vi "Init tree for error log.vi"(8 "error in (no error)":errorcluster, 9 "Test Log(Schema)":string=" edcu_48v_thermal_endurance_test_dv_28_10_2024_19_48_44.error_log" caption="Test Log", 11 "TreeControl in":refnum<vi>) -> (0 "error out":errorcluster)   [LabVIEW 2023, in "Data Analysis.lvlib"]
uses:
  Data Analysis.lvlib
  HardwareAbstractionLayer_LVOOP/Database/Database.lvclass
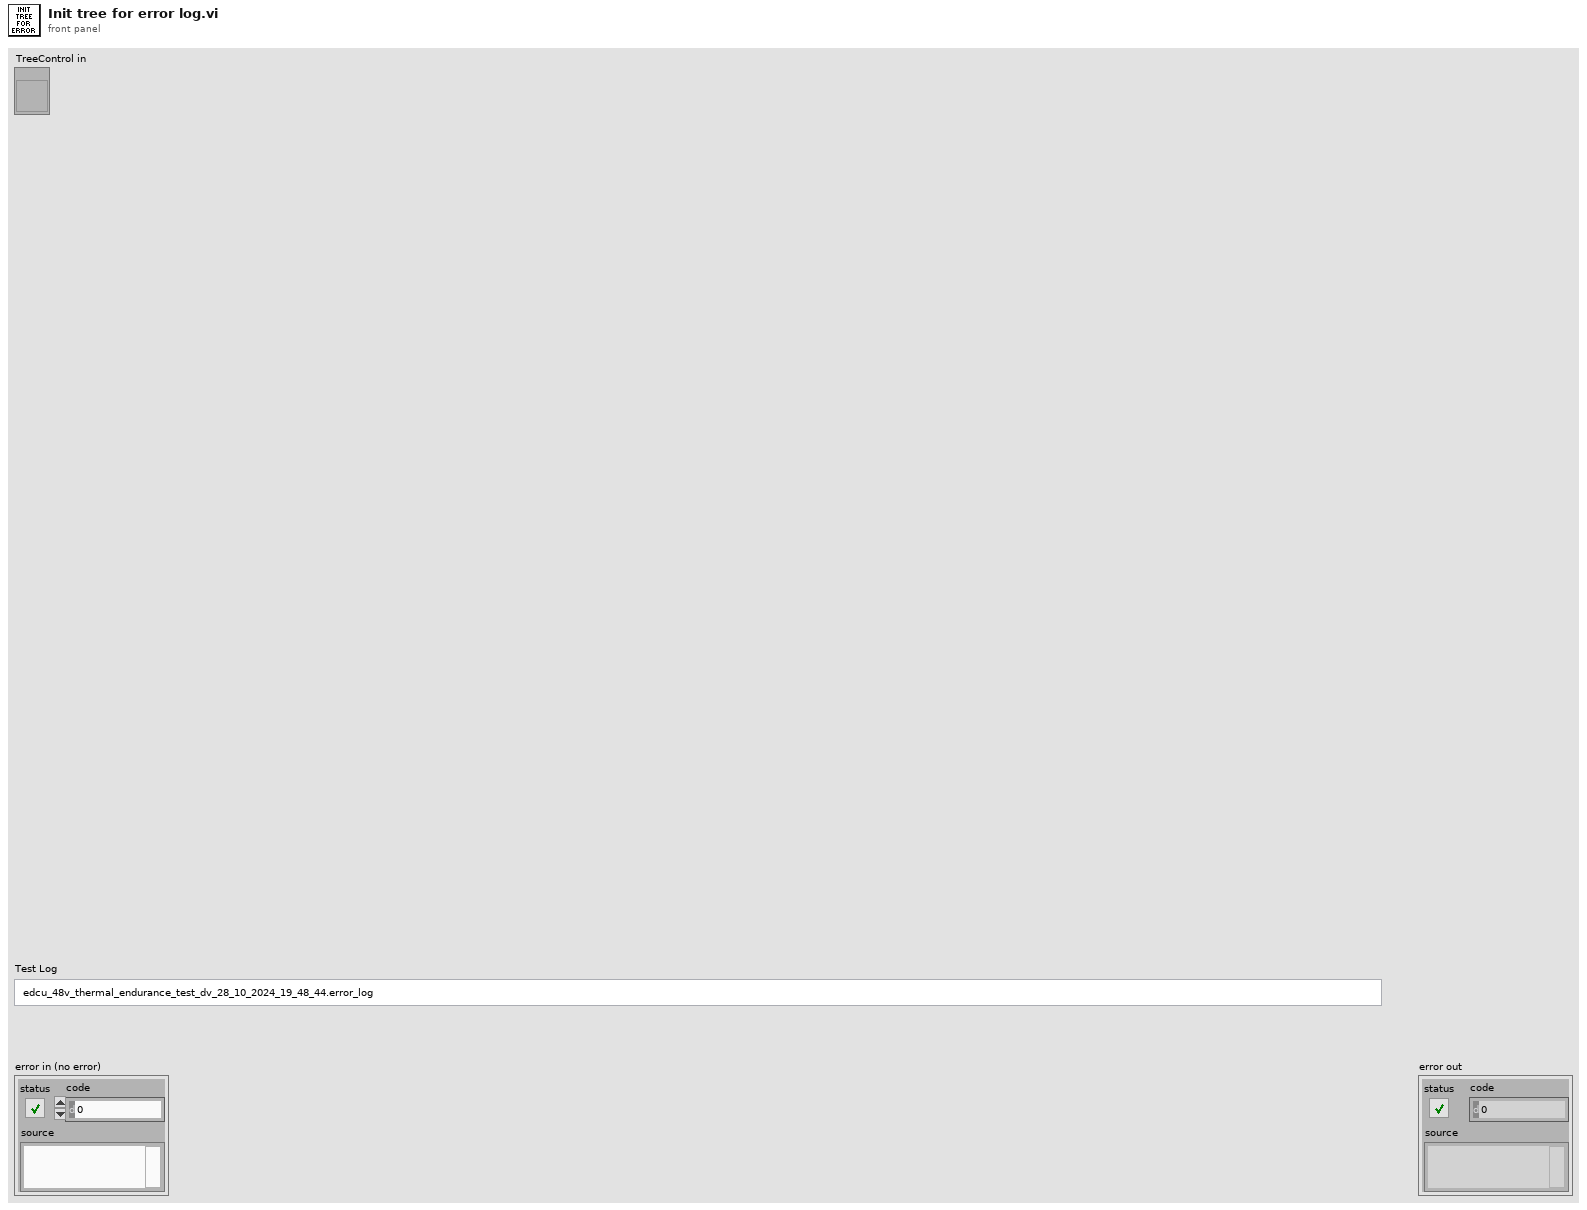
[diagram p1: front panel]
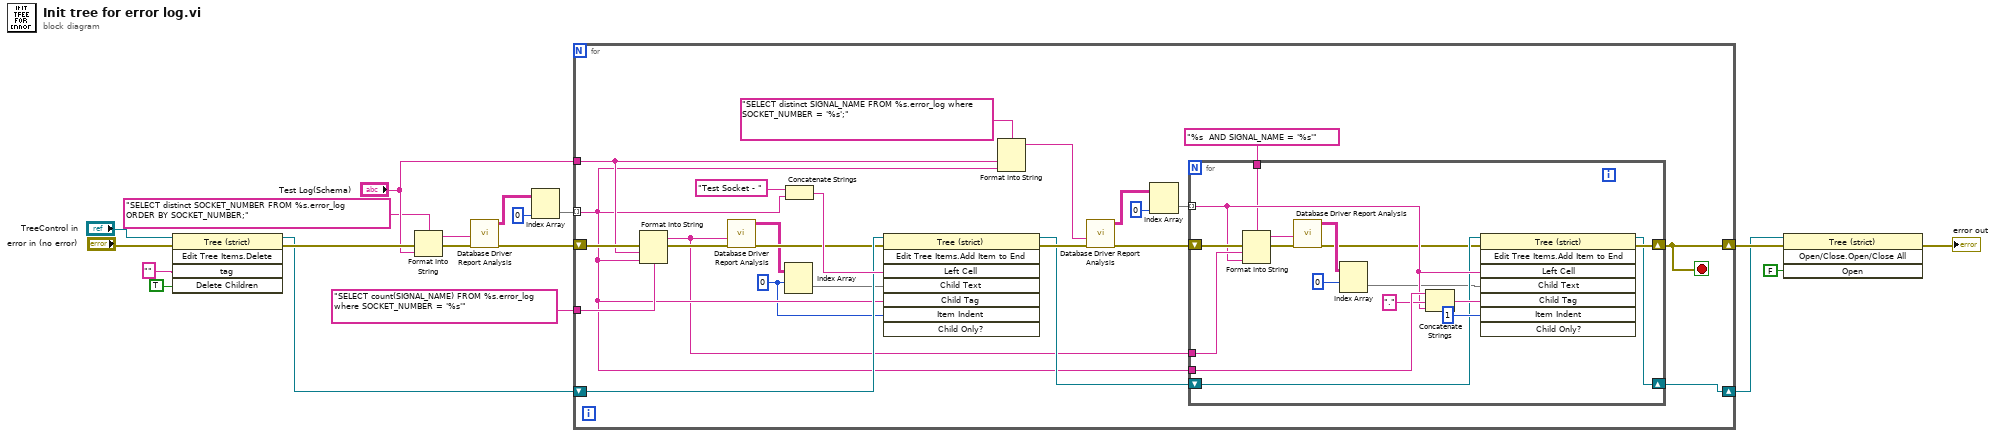
[diagram p0: block diagram]
diagram:
  n1 = invoke on="Invoke Node" class="Tree (strict)" method="Edit Tree Items.Delete"(reference="TreeControl in", error in="error in (no error)", "tag"="" ("Tag"), "Delete Children"=TRUE ("Delete Children?")) -> (reference out=w1:refnum<vi>, error out=w16:errorcluster)  [unwired: 1 in, 3 out]
  n2 = Format Into String(format string="SELECT distinct SOCKET_NUMBER FROM %s.error_log ORDER BY SOCKET_NUMBER;" ("SQL query"), error in=w16, "Test Log(Schema)") -> (resulting string=w12:string, error out=w17:errorcluster)  [unwired: 1 in]
  n3 = call "Database Driver Report Analysis.vi"("error in"=w17, "SQL query"=w12) -> ("error out"=w8:errorcluster, "data"=w9:string[][])  [unwired: 6 in, 2 out]
  n4 = Index Array(array=w9, index (col)=0 ("disabled index (col)")) -> (element=w10:string[])  [unwired: 1 in]
  n5 = for {
    tunnel: w10 -> [w25] mode=indexing
    shift-right: [w41] -> w18
    shift-left: w8 -> [w29]
    tunnel: "Test Log(Schema)" -> [w26]
    shift-right: [w31] -> w3
    shift-left: w1 -> [w33]
    tunnel: "SELECT count(SIGNAL_NAME) FROM %s.error_log where SOCKET_NUMBER = '%s'" ("SQL query") -> [w27]
    stop <- w41 stop-if-true
    w22 = 0 ("index (row)")
    n6 = Format Into String(format string=w27, error in=w29, w26, w25) -> (resulting string=w21:string, error out=w28:errorcluster)  [unwired: 1 in]
    n7 = call "Database Driver Report Analysis.vi"("error in"=w28, "SQL query"=w21) -> ("error out"=w30:errorcluster, "data"=w24:string[][])  [unwired: 6 in, 2 out]
    n8 = Index Array(array=w24, index (row)=w22) -> (element=w23:string[])  [unwired: 1 in]
    n9 = Concatenate Strings("Test Socket - " ("element"), w25) -> (w42:string)
    n10 = invoke on="Invoke Node" class="Tree (strict)" method="Edit Tree Items.Add Item to End"(reference=w33, error in=w30, "Left Cell"=w42, "Child Text"=w23, "Child Tag"=w25, "Item Indent"=w22) -> (reference out=w32:refnum<vi>, error out=w40:errorcluster)  [unwired: 2 in, 6 out]
    n11 = Format Into String(format string="SELECT distinct SIGNAL_NAME FROM %s.error_log where SOCKET_NUMBER = '%s';" ("SQL query"), w26, w25) -> (resulting string=w37:string)  [unwired: 2 in, 1 out]
    n12 = call "Database Driver Report Analysis.vi"("error in"=w40, "SQL query"=w37) -> ("error out"=w39:errorcluster, "data"=w35:string[][])  [unwired: 6 in, 2 out]
    n13 = Index Array(array=w35, index (col)=0 ("disabled index (col)")) -> (element=w34:string[])  [unwired: 1 in]
    n14 = for {
      shift-right: [w60] -> w41
      shift-left: w39 -> [w54]
      tunnel: w34 -> [w52] mode=indexing
      tunnel: w25 -> [w58]
      shift-right: [w55] -> w31
      shift-left: w32 -> [w50]
      tunnel: w21 -> [w53]
      tunnel: "%s  AND SIGNAL_NAME = '%s'" ("format string") -> [w51]
      n15 = Format Into String(format string=w51, error in=w54, w53, w52) -> (resulting string=w44:string, error out=w47:errorcluster)  [unwired: 1 in]
      n16 = call "Database Driver Report Analysis.vi"("error in"=w47, "SQL query"=w44) -> ("error out"=w46:errorcluster, "data"=w49:string[][])  [unwired: 6 in, 2 out]
      n17 = Index Array(array=w49, index (row)=0) -> (element=w45:string[])  [unwired: 1 in]
      n18 = Concatenate Strings(w58, "." ("string"), w52) -> (w56:string)
      n19 = invoke on="Invoke Node" class="Tree (strict)" method="Edit Tree Items.Add Item to End"(reference=w50, error in=w46, "Left Cell"=w52, "Child Text"=w45, "Child Tag"=w56, "Item Indent"=1 ("New Item Indentation")) -> (reference out=w55:refnum<vi>, error out=w60:errorcluster)  [unwired: 2 in, 6 out]
    }
  }
  n20 = invoke on="Invoke Node" class="Tree (strict)" method="Open/Close.Open/Close All"(reference=w3, error in=w18, "Open"=FALSE ("Open?")) -> (error out=→"error out":errorcluster)  [unwired: 1 in, 3 out]
